vi "Read Handle Cluster.vi"(8 "error in (no error)":errorcluster, 11 "Initialize_card in":refnum<class "Initialize_card.lvclass">) -> (0 "error out":errorcluster, 2 "Handle Cluster":T1, 3 "Initialize_card out":refnum<class "Initialize_card.lvclass">)   [LabVIEW 2015, in "Initialize_card.lvclass"]
uses:
  Initialize_card.lvclass
  Initialize_card.lvclass/Initialize_card.ctl
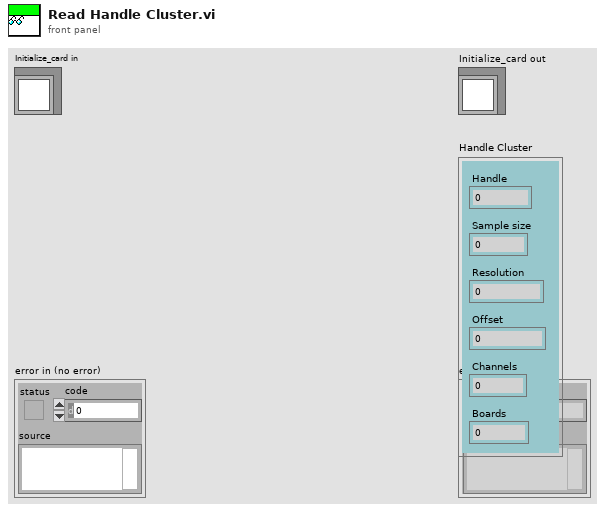
[diagram p1: front panel]
types:
  T1 = cluster{"Handle":u32, "Sample size":u32, "Resolution":i32, "Offset":i32, "Channels":u32, "Boards":u32}
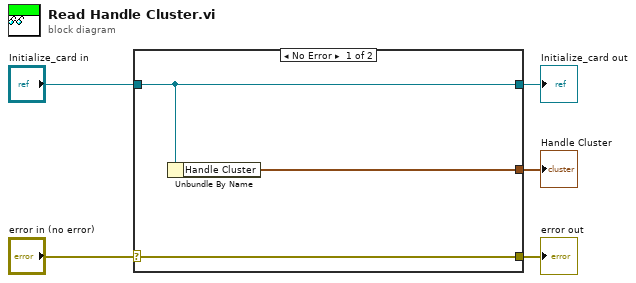
[diagram p0: block diagram]
diagram:
  n1 = case shown="No Error" "error in (no error)" {
    selector: "error in (no error)" -> [w8 w9]
    tunnel: [w8 w9] -> w4
    tunnel: [w7 w10] -> w2
    tunnel: "Initialize_card in" -> [w7 w10]
    tunnel: [w6 _] -> w1
    frame No Error {
      n2 = Unbundle By Name(w7) -> ("Handle Cluster"=w6:T1)
    }
    frame Error {
    }
  }
  "error out" <- w4
  "Initialize_card out" <- w2
  "Handle Cluster" <- w1
